vi "Get Server DLL Path.vi"() -> (0 "Server dll path":path)   [LabVIEW 2024, in "grpc-lvsupport.lvlib"]
uses:
  grpc-lvsupport.lvlib
  <vilib>/Utility/LVLibp/NI_PackedLibraryUtility.lvlib
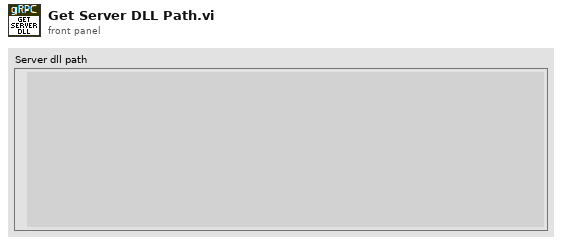
[diagram p1: front panel]
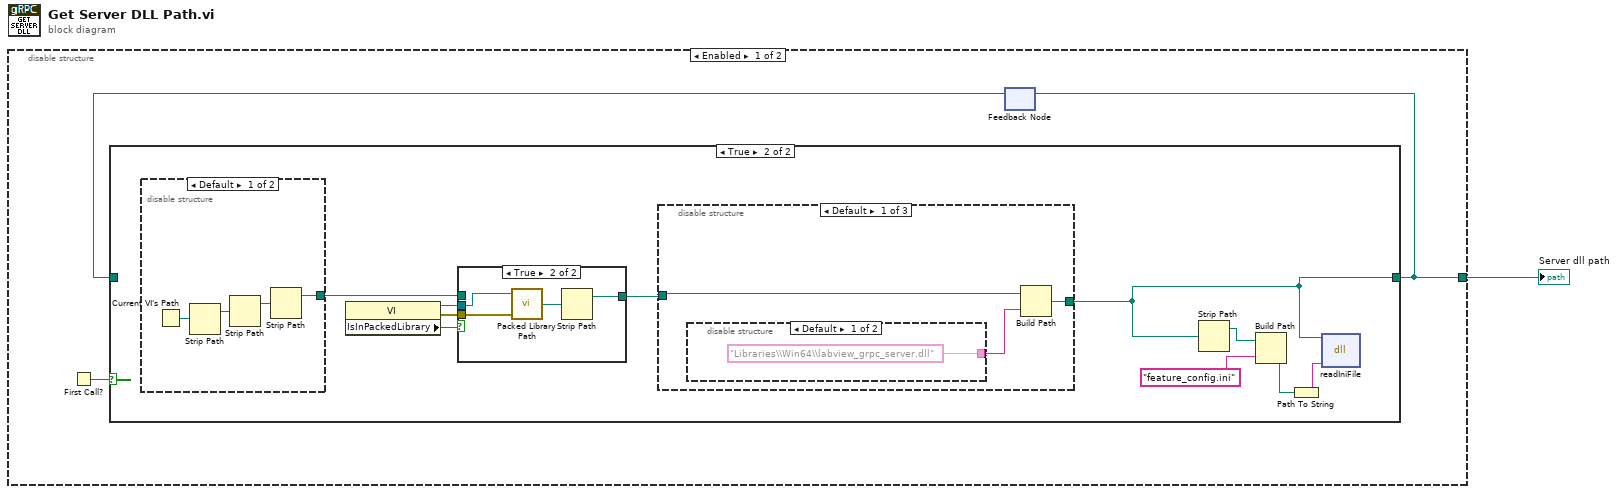
[diagram p0: block diagram]
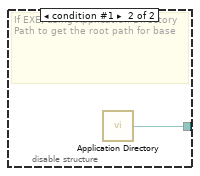
[diagram p4: hidden frame]
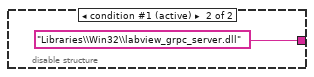
[diagram p5: hidden frame]
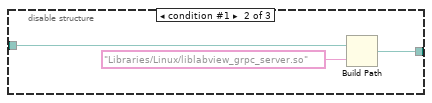
[diagram p6: hidden frame]
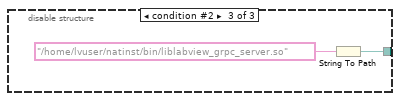
[diagram p7: hidden frame]
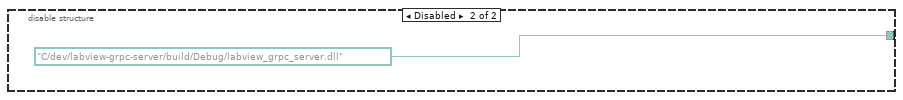
[diagram p8: hidden frame]
diagram:
  n1 = disable-structure shown="Enabled" {
    disable-tunnel: [w3 path "C:/dev/labview-grpc-server/build/Debug/labview_grpc_server.dll" ("Server dll path")] -> w1
    frame Enabled {
      n2 = First Call?() -> (First Call?: T/F=w4:bool)
      n3 = feedback #1() -> (w2:path)  [unwired: 1 in]
      n4 = case shown="True" w4 {
        tunnel: [w5 w6] -> w3
        tunnel: w2 -> [w5 _]
        frame False {
        }
        frame True {
          n5 = disable-structure shown="Default" {
            disable-tunnel: [w21 w25] -> w12
            frame condition #0 (active) {
              n6 = Current VI's Path() -> (path=w23:path)
              n7 = Strip Path(path=w23) -> (stripped path=w24:path)  [unwired: 1 out]
              n8 = Strip Path(path=w24) -> (stripped path=w22:path)  [unwired: 1 out]
              n9 = Strip Path(path=w22) -> (stripped path=w21:path)  [unwired: 1 out]
            }
            frame condition #1 {
              # "If EXE, using Application Directory Path to get the root path for base"
              n10 = call <vilib>:"Application Directory.vi"() -> ("Application Directory"=w25:path)
            }
          }
          n11 = property class="VI"() -> (reference out=w14:refnum<vi>, error out=w15:errorcluster, "IsInPackedLibrary"=w13:bool)  [unwired: 2 in]
          n12 = case shown="True" w13 {
            tunnel: w14 -> [_ w20]
            tunnel: w15 -> [_ w19]
            tunnel: [w16 w18] -> w11
            tunnel: w12 -> [w16 _]
            frame False {
            }
            frame True {
              n13 = call <vilib>:"Packed Library Path.vi"("error in (no error)"=w19, "vi reference"=w20) -> ("packed library path"=w17:path)  [unwired: 1 in, 2 out]
              n14 = Strip Path(path=w17) -> (stripped path=w18:path)  [unwired: 1 out]
            }
          }
          n15 = disable-structure shown="Default" {
            disable-tunnel: w11 -> [w26 w33 _]
            disable-tunnel: [w27 w32 w34] -> w6
            frame condition #0 (active) {
              n16 = disable-structure shown="Default" {
                disable-tunnel: ["Libraries\\Win64\\labview_grpc_server.dll" ("name or relative path") "Libraries\\Win32\\labview_grpc_server.dll" ("name or relative path")] -> w28
                frame condition #0 {
                }
                frame condition #1 (active) {
                }
              }
              n17 = Build Path(base path=w26, name or relative path=w28) -> (appended path=w27:path)
            }
            frame condition #1 {
              n18 = Build Path(base path=w33, name or relative path="Libraries/Linux/liblabview_grpc_server.so") -> (appended path=w32:path)
            }
            frame condition #2 {
              n19 = String To Path(string="/home/lvuser/natinst/bin/liblabview_grpc_server.so" ("name or relative path")) -> (path=w34:path)
            }
          }
          n20 = Strip Path(path=w6) -> (stripped path=w10:path)  [unwired: 1 out]
          n21 = Build Path(base path=w10, name or relative path="feature_config.ini") -> (appended path=w8:path)
          n22 = Path To String(path=w8) -> (string=w7:string)
          n23 = dll-call lib="?" fn="readIniFile"(path in=w6, "filePath"=w7) -> ()  [unwired: 4 in, 2 out]
        }
      }
      n24 = feedback-in #1(w3) -> ()
    }
    frame Disabled {
    }
  }
  "Server dll path" <- w1
